vi "SRSRampWrite.vi"(1 "GPIB Address":i32, 2 "error in":errorcluster, 3 "XY Vector":dbl[][](array[numeric]) format="%.3p", 4 "time resolution":dbl=0.00015 format="%.3p", 5 "Amplitude":dbl=2.9999326394505683 format="%_5p") -> (0 "error out":errorcluster)   [LabVIEW 2013, in "SubVIs.lvlib"]
uses:
  SubVIs.lvlib
panel:
  out "points":i16
  out "Output Array":i16[](array[numeric])=[0, 0, 0, 0, 0, 0, 0, 0, 0, 0, 0, 0, 0, 0, 0, 0, 0, 0, 0, 0, 0, 0, 0, 0, 0, 0, 0, 0, 0, 0, 0, 0, 0, 0, 0, 0, 0, 0, 0, 0, 0, 0, 0, 0, 0, 0, 0, 0, 0, 0, 0, 0, 0, 0, 0, 0, 0, 0, 0, 0, 0, 0, 0, 0, 0, 0, 0, 0, 0, 0, 0, 0, 0, 0, 0, 0, 0, 0, 0, 0, 0, 0, 0, 0, 0, 0, 0, 0, 0, 0, 0, 0, 0, 0, 0, 0, 0, 0, 0, 0, 0, 0, 1, 0, 1, 0, 1, 0, 1, 0, 1, 0, 1, 0, 1, 0, 1, 0, 1, 0, 1, 1, 1, 1, 1, 1, 1, 2, 1, 3, 1, 4, 1, 6, 1, 9, 1, 12, 1, 17, 1, 23, 1, 31, 1, 41, 1, 53, 1, 70, 1, 90, 1, 115, 1, 145, 1, 182, 1, 226, 1, 277, 1, 337, 1, 405, 1, 483, 1, 569, 1, 665, 1, 768, 1, 879, 1, 996, 1, 1118, 1, 1242, 1, 1365, 1, 1486, 1, 1602, 1, 1710, 1, 1806, 1, 1890, 1, 1957, 1, 2006, 1, 2037, 1, 2047, 1, 2047, 1, 2037, 1, 2006, 1, 1957, 1, 1890, 1, 1806, 1, 1710, 1, 1602, 1, 1486, 1, 1365, 1, 1242, 1, 1118, 1, 996, 1, 879, 1, 768, 1, 665, 1, 569, 1, 483, 1, 405, 1, 337, 1, 277, 1, 226, 1, 182, 1, 145, 1, 115, 1, 90, 1, 70, 1, 53, 1, 41, 1, 31, 1, 23, 1, 17, 1, 12, 1, 9, 1, 6, 1, 4, 1, 3, 1, 2, 1, 1, 1, 1, 2, 1, 2, 0, 2, 0, 2, 0, 2, 0, 2, 0, 2, 0, 2, 0, 2, 0, 2, 0, 2, 0, 2, 0, 2, 0, 2, 0, 2, 0, 2, 0, 2, 0, 2, 0, 2, 0, 2, 0, 2, 0, 2, 0, 2, 0, 2, 0, 2, 0, 2, 0, 2, 0, 2, 0, 2, 0, 2, 0, 2, 0, 2, 0, 2, 0, 2, 0, 2, 0, 2, 0, 2, 0, 2, 0, 2, 0, 2, 0, 2, 0, 2, 0, 2, 0, 2, 0, 2, 0, 2, 0, 2, 0, 2, 0, 2, 0, 2, 0, 2, 0, 2, 0, 2, 0, 2, 0, 2, 0, 2, 0, 2, 0, 2, 0, 2, 0, 2, 0, 2, 0, -11970]
  # "Time (s)"
  # "Output (fraction)"
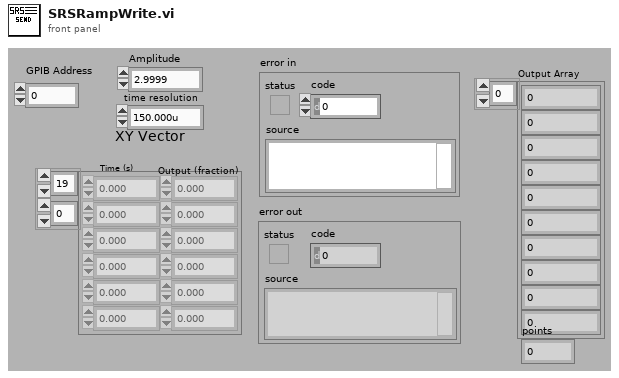
[diagram p1: front panel]
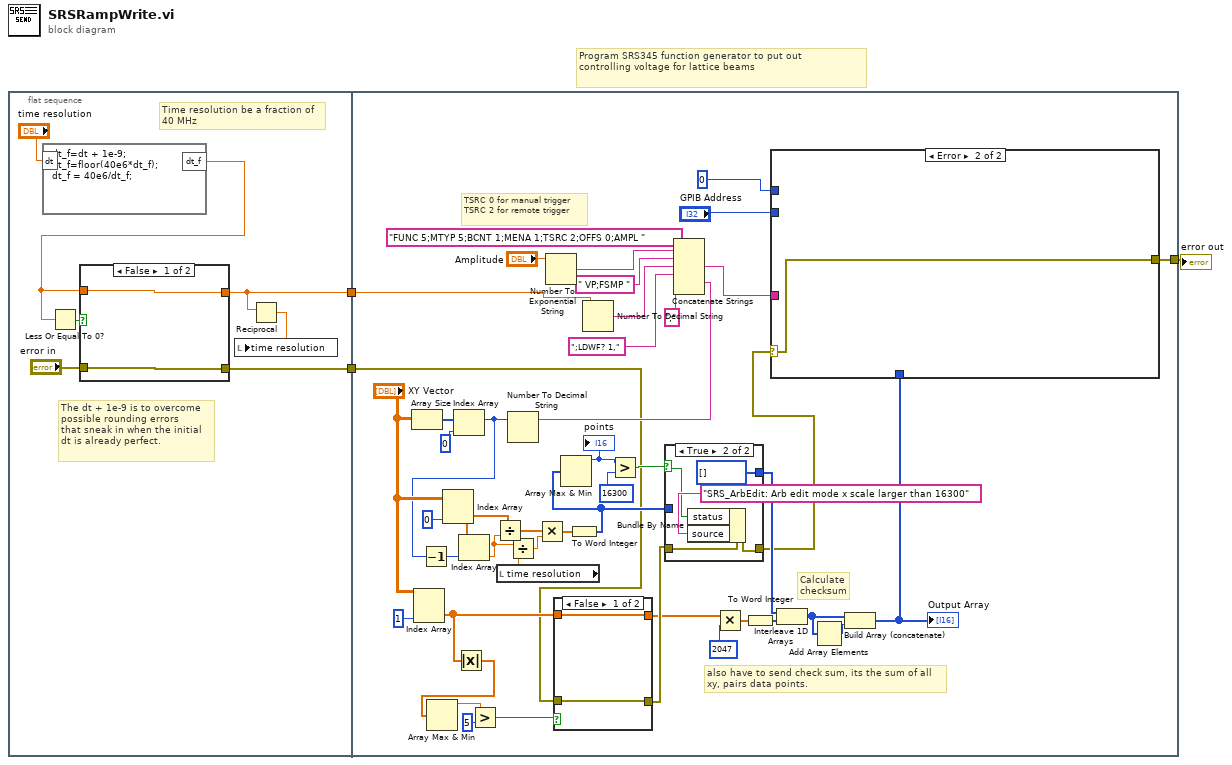
[diagram p0: block diagram]
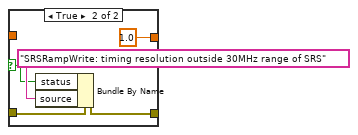
[diagram p2: hidden frame]
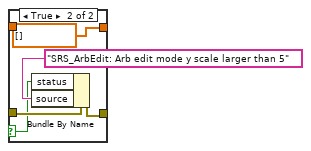
[diagram p3: hidden frame]
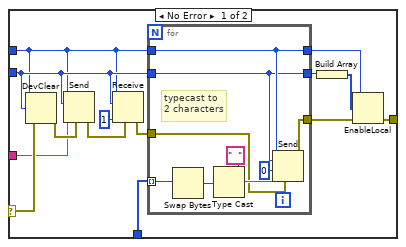
[diagram p4: hidden frame]
diagram:
  # "Program SRS345 function generator to put out\ncontrolling voltage for lattice beams"
  n1 = flat-sequence {
    tunnel: [w9] -> w2
    tunnel: [w5] -> w1
    tunnel: [w23] -> w3
    tunnel: w2 -> [w21]
    tunnel: w1 -> [w20]
    frame #0 {
      # "The dt + 1e-9 is to overcome\npossible rounding errors\nthat sneak in when the initial\ndt is already perfect."
      # "Time resolution be a fraction of \n40 MHz"
      n2 = formula code="dt_f=dt + 1e-9;\ndt_f=floor(40e6*dt_f);\ndt_f = 40e6/dt_f;"("dt"="time resolution") -> ("dt_f"=w6:dbl)
      n3 = Less Or Equal To 0?(x=w6) -> (x <= 0?=w7:bool)
      n4 = case shown="False" w7 {
        selector: w7 -> [_ w15]
        tunnel: "error in" -> [w12 w17]
        tunnel: [w12 w14] -> w9
        tunnel: [w11 1.0] -> w5
        tunnel: w6 -> [w11 _]
        frame False {
        }
        frame True {
          n5 = Bundle By Name(cluster=w17, "status"=w15, "source"="SRSRampWrite: timing resolution outside 30MHz range of SRS") -> (w14:errorcluster)
        }
      }
      n6 = Reciprocal(x=w5) -> (1/x=w4:dbl)
      n7 = local write "time resolution"(w4) -> ()
    }
    frame #1 {
      # "TSRC 0 for manual trigger\nTSRC 2 for remote trigger"
      # "Calculate\nchecksum"
      # "also have to send check sum, its the sum of all \nxy, pairs data points."
      n8 = Array Size(array="XY Vector") -> (size(s)=w46:i32[])
      n9 = Index Array(array="XY Vector", index (col)=1 ("Disabled Index (col)")) -> (element=w28:dbl[])  [unwired: 1 in]
      n10 = Index Array(array="XY Vector", index (col)=0 ("Disabled Index (col)")) -> (element=w45:dbl[])  [unwired: 1 in]
      n11 = Index Array(array=w46, index=0 ("Index")) -> (element=w35:i32)
      n12 = Decrement(x=w35) -> (x-1=w36:i32)
      n13 = Absolute Value(x=w28) -> (abs(x)=w18:dbl[])
      n14 = Array Max & Min(array=w18) -> (max value=w26:dbl)  [unwired: 3 out]
      n15 = Index Array(array=w45, index=w36) -> (element=w34:dbl)
      n16 = Greater?(x=w26, y=5) -> (0:w25:bool)
      n17 = Divide(x=w45, y=w34) -> (x/y=w44:dbl[])
      n18 = local read "time resolution"() -> (w33:dbl)
      n19 = Number To Decimal String(number=w35) -> (decimal integer string=w51:string)  [unwired: 1 out]
      n20 = Divide(x=w34, y=w33) -> (x/y=w32:dbl)
      n21 = Multiply(x=w44, y=w32) -> (x*y=w42:dbl[])
      n22 = Number To Exponential String(number="Amplitude") -> (E-format string=w50:string)  [unwired: 3 out]
      n23 = case shown="False" w25 {
        selector: w25 -> [_ w68]
        tunnel: w21 -> [w65 w70]
        tunnel: [w65 w67] -> w30
        tunnel: w28 -> [w64 _]
        tunnel: [w64 dbl[] [] ("XY Vector")] -> w29
        frame False {
        }
        frame True {
          n24 = Bundle By Name(cluster=w70, "status"=w68, "source"="SRS_ArbEdit: Arb edit mode y scale larger than 5") -> (w67:errorcluster)
        }
      }
      n25 = To Word Integer(number=w42) -> (16bit integer=w39:i16[])
      n26 = Array Max & Min(array=w39) -> (max value=w41:i16)  [unwired: 3 out]
      "points" <- w41
      n27 = Number To Decimal String(number=w20) -> (decimal integer string=w61:string)  [unwired: 1 out]
      n28 = Greater?(x=w41, y=16300) -> (0:w43:bool)
      n29 = case shown="True" w43 {
        selector: w43 -> [_ w98]
        tunnel: w30 -> [w95 w100]
        tunnel: [w95 w97] -> w22
        tunnel: [w94 i16[] []] -> w38
        tunnel: w39 -> [w94 _]
        frame False {
        }
        frame True {
          n30 = Bundle By Name(cluster=w100, "status"=w98, "source"="SRS_ArbEdit: Arb edit mode x scale larger than 16300") -> (w97:errorcluster)
        }
      }
      n31 = Concatenate Strings("FUNC 5;MTYP 5;BCNT 1;MENA 1;TSRC 2;OFFS 0;AMPL ", w50, " VP;FSMP ", w61, ";LDWF? 1,", w51, ";") -> (w62:string)
      n32 = Multiply(x=w29, y=2047) -> (x*y=w56:dbl[])
      n33 = To Word Integer(number=w56) -> (16bit integer=w49:i16[])
      n34 = Interleave 1D Arrays(w38, w49) -> (w55:i16[])
      n35 = Add Array Elements(numeric array=w55) -> (sum=w54:i16)
      n36 = Build Array (concatenate)(w55, w54) -> (w53:i16[])
      "Output Array" <- w53
      n37 = case shown="Error" w22 {
        selector: w22 -> [w72 w93]
        tunnel: w62 -> [w71 _]
        tunnel: [w76 w93] -> w23
        tunnel: "GPIB Address" -> [w75 _]
        tunnel: w53 -> [w81 _]
        tunnel: 0 ("bus") -> [w73 _]
        frame No Error {
          n38 = DevClear(2:w72, 3:w75, 4:w73) -> (0:w74:errorcluster)  [unwired: 1 out]
          n39 = Send(0:w73, 2:w75, 4:w74, 5:w71) -> (8:w82:errorcluster)  [unwired: 3 out]
          n40 = Receive(4:w82, 6:1 ("count"), 8:w75, 9:w73) -> (0:w80:errorcluster)  [unwired: 4 out]
          n41 = for {
            tunnel: w81 -> [w90] mode=indexing
            tunnel: [w91] -> w76
            tunnel: w80 -> [w86]
            tunnel: w73 -> [w85]
            tunnel: w75 -> [w84]
            tunnel: [w85] -> w78
            tunnel: [w84] -> w77
            # "typecast to\n2 characters"
            n42 = Swap Bytes(anything=w90) -> (byte swapped=w89:i16)
            n43 = Type Cast(type="  ", x=w89) -> (*(type *) &x=w87:string)
            n44 = Send(0:w85, 2:w84, 3:i16 0 ("mode"), 4:w86, 5:w87) -> (8:w91:errorcluster)  [unwired: 2 out]
          }
          n45 = Build Array(w77) -> (w79:i32[])
          n46 = EnableLocal(3:w79, 4:w78) -> ()  [unwired: 1 in, 2 out]
        }
        frame Error {
        }
      }
    }
  }
  "error out" <- w3
